vi "Practica3_try2.vi"() -> ()   [LabVIEW 2018]
uses:
  <vilib>/MakerHub/LINX/Public/Peripherals/PWM/PWM Set Duty Cycle 1 Chan.vi
  <vilib>/MakerHub/LINX/Public/Peripherals/Analog/Analog Read 1 Chan.vi
  <vilib>/MakerHub/LINX/Public/Peripherals/Analog/Analog Read N Chans.vi
  <vilib>/MakerHub/LINX/Private/Local IO/LinxAnalogRead.vi
  <vilib>/MakerHub/LINX/Public/Utilities/Check Channel.vi
  <vilib>/MakerHub/LINX/Public/Utilities/Open Serial.vi
  <vilib>/MakerHub/LINX/Public/Sensors/Temperature/TMP3x/TMP35.vi
  <vilib>/MakerHub/LINX/Public/Peripherals/PWM/PWM Set Duty Cycle N Chans.vi
  <vilib>/MakerHub/LINX/Private/Utilties/Generate Error.vi
  <vilib>/MakerHub/LINX/LMH-LINX.lvlib
  <vilib>/MakerHub/LINX/Public/Sensors/Temperature/TMP3x/TMP3x.lvlib
  <vilib>/ptbypt/NI_PtbyPt.lvlib
panel:
  in  "y 3":errorcluster
  in  "y 2":errorcluster
  out "Boolean":bool
  in  "Serial Port":refnum<visa-resource-name>="N/A"
  in  "Temperatura limite":dbl
  out "Thermometer":dbl(slide) scale=0.0..100.0
  in  "y":errorcluster
  out "Color Box 2":u32(colorbox)
  in  "intensidd verde":dbl=0.3
  in  "Temperatur optima(led azul)":dbl=0.25 format="%#_13g"
  in  "stop":bool
  in  "hall":bool
  in  "lm35":bool
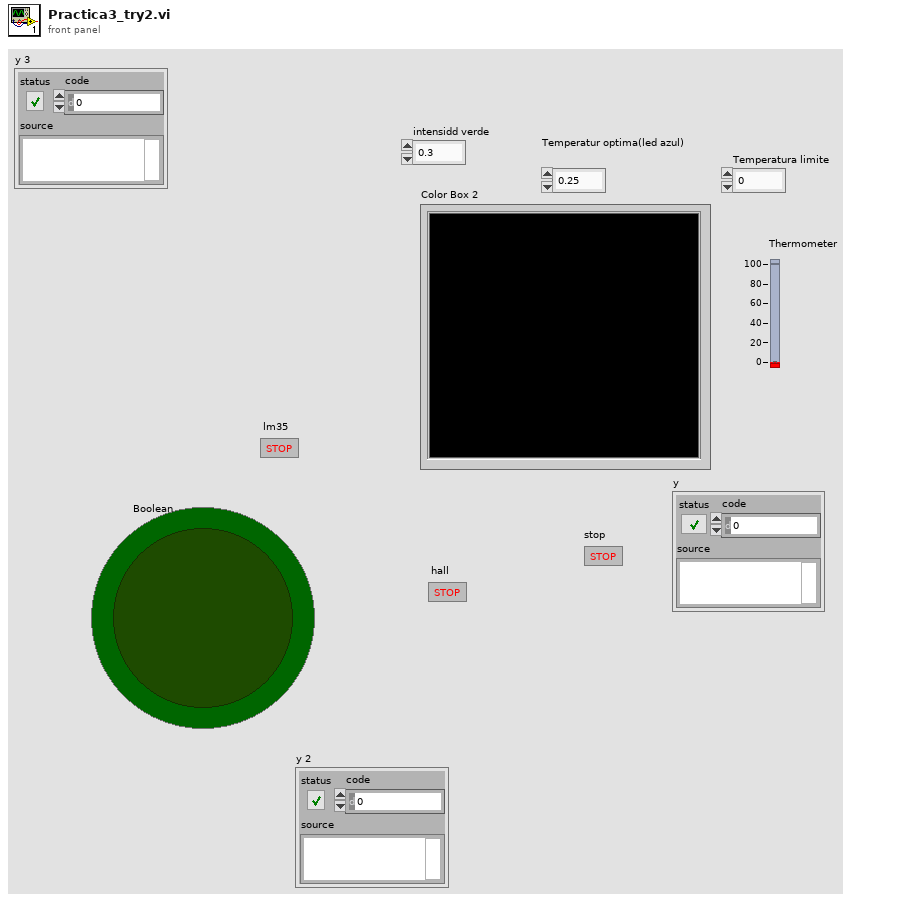
[diagram p1: front panel]
types:
  T1 = typedef "LMH-LINX.lvlib/LINX Ref.ctl" = cluster{"IO":T2, "Interface":T3, "LINX Device Config":T4}
  T2 = typedef "LMH-LINX.lvlib/Platform.ctl" = enum16{"Remote", "Local"}
  T3 = typedef "LMH-LINX.lvlib/Interface.ctl" = enum16{"Serial", "TCP"}
  T4 = typedef "LMH-LINX.lvlib/Device.lvlib/LINX Device Config.ctl" = cluster{"Interface":T3, "COM Port":refnum<visa-resource-name>, "TCP Configuration":T5, "Device Family":u8, "Device ID":u8, "Device Name":string, "TCP Ref":refnum<k5>, "Channels":T6}
  T5 = typedef "LMH-LINX.lvlib/Device.lvlib/TCP Config.ctl" = cluster{"IP Address":string, "Port":u16}
  T6 = typedef "LMH-LINX.lvlib/Channels.ctl" = cluster{"DI":u8[], "DO":u8[], "AI":u8[], "AO":u8[], "PWM":u8[], "QE":u8[], "UART":u8[], "I2C 2":u8[], "SPI":u8[], "CAN":u8[], "Servo":u8[], "AI Ref (V)":dbl, "AI Resolution (Bits)":u8, "AO Ref (V)":dbl, "AO Resolution (Bits)":u8}
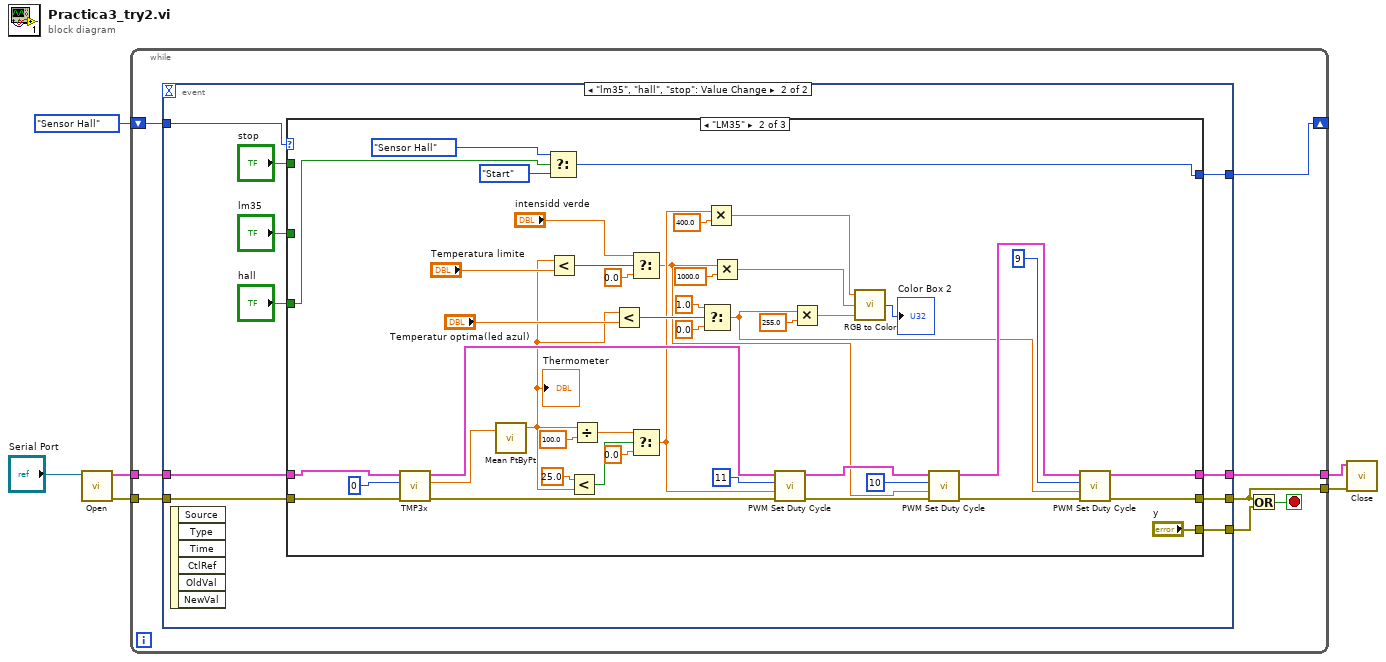
[diagram p0: block diagram]
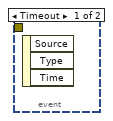
[diagram p2: hidden frame]
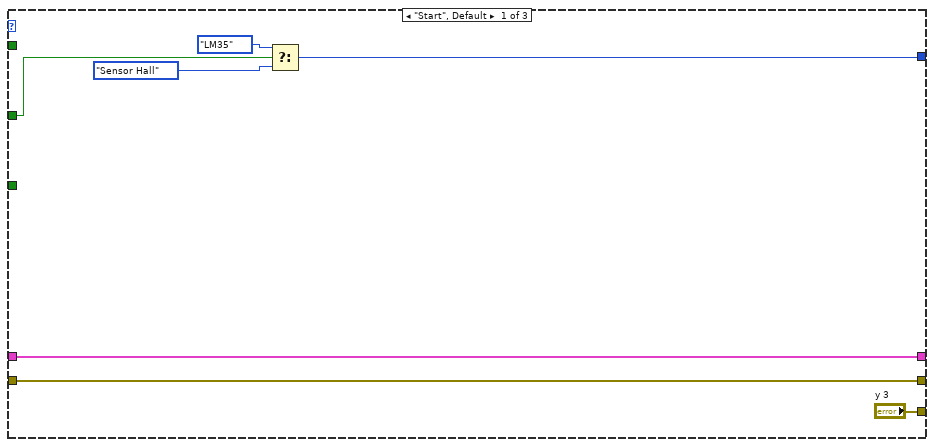
[diagram p3: hidden frame]
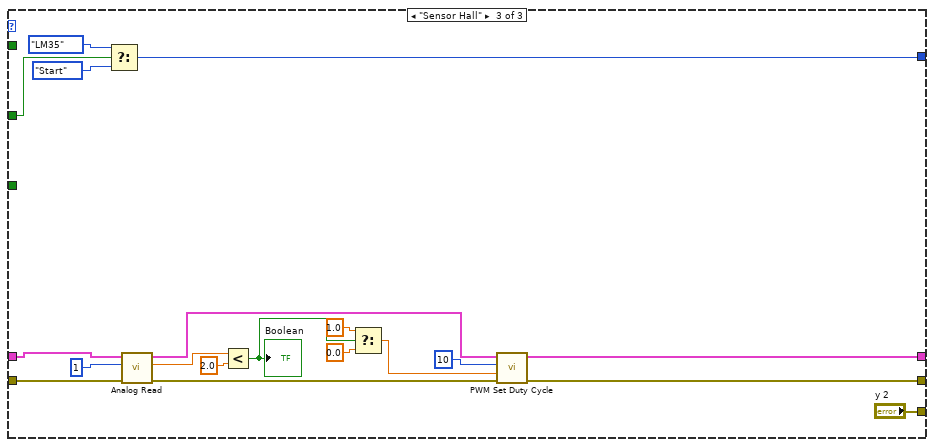
[diagram p4: hidden frame]
diagram:
  n1 = call-poly <vilib>:"Open.vi"("Serial Port"="Serial Port") -> ("Error Out"=w3:errorcluster, "LINX Resource"=w4:T1)  [unwired: 8 in, 1 out]
  n2 = while {
    shift-right: [w14] -> _
    shift-left: enum16{"Start", "LM35", "Sensor Hall"}."Sensor Hall" -> [w13]
    tunnel: w4 -> [w12]
    tunnel: w3 -> [w11]
    tunnel: [w10] -> w2
    tunnel: [w8] -> w1
    stop <- w9 stop-if-true
    n3 = event shown="[1] \"lm35\", \"hall\", \"stop\": Value Change" {
      selector: _ -> [_ _]
      dyn-events: _ -> [_ _]
      timeout: _ -> [_ _]
      tunnel: w13 -> [_ w24]
      tunnel: [_ w20] -> w14
      tunnel: w12 -> [_ w19]
      tunnel: w11 -> [_ w18]
      tunnel: [_ w17] -> w10
      tunnel: [_ w16] -> w8
      tunnel: [_ w15] -> w7
      event Timeout {
        n4 = event-data() -> ()  [unwired: 1 in, 3 out]
      }
      event "lm35", "hall", "stop": Value Change {
        n5 = event-data() -> ()  [unwired: 1 in, 6 out]
        n6 = case shown="\"LM35\"" w24 {
          tunnel: "stop" -> [_ _ _]
          tunnel: "lm35" -> [w28 _ w92]
          tunnel: "hall" -> [_ w75 _]
          tunnel: [w30 w73 w91] -> w20
          tunnel: w19 -> [w27 w36 w77]
          tunnel: w18 -> [w26 w35 w76]
          tunnel: [w27 w34 w80] -> w17
          tunnel: [w26 w33 w79] -> w16
          tunnel: ["y 3" "y" "y 2"] -> w15
          frame "Start", Default {
            n7 = Select(t=enum16{"Start", "LM35", "Sensor Hall"}."LM35", s=w28, f=enum16{"Start", "LM35", "Sensor Hall"}."Sensor Hall") -> (s? t:f=w30:enum16{"Start", "LM35", "Sensor Hall"})
          }
          frame "LM35" {
            n8 = call-poly <vilib>:"TMP3x.vi"("Error In"=w35, "Analog Channel"=u8 0, "LINX Resource"=w36) -> ("Error Out"=w61:errorcluster, "Temp C"=w43:dbl, "LINX Resource"=w60:T1)  [unwired: 6 in]
            n9 = call <vilib>:"Mean PtByPt.vi"("x"=w43) -> ("mean"=w37:dbl)  [unwired: 3 in, 1 out]
            "Thermometer" <- w37
            n10 = Select(t=enum16{"Start", "LM35", "Sensor Hall"}."Sensor Hall", s=w75, f=enum16{"Start", "LM35", "Sensor Hall"}."Start") -> (s? t:f=w73:enum16{"Start", "LM35", "Sensor Hall"})
            n11 = Less?(x=w37, y="Temperatura limite") -> (x < y?=w42:bool)
            n12 = Less?(x=25.0, y=w37) -> (x < y?=w62:bool)
            n13 = Divide(x=w37, y=100.0) -> (x/y=w57:dbl)
            n14 = Less?(x=w37, y="Temperatur optima(led azul)") -> (x < y?=w66:bool)
            n15 = Select(t="intensidd verde", s=w42, f=0.0) -> (s? t:f=w41:dbl)
            n16 = Select(t=w57, s=w62, f=0.0) -> (s? t:f=w52:dbl)
            n17 = Select(t=1.0, s=w66, f=0.0) -> (s? t:f=w44:dbl)
            n18 = Multiply(x=w52, y=400.0) -> (x*y=w47:dbl)
            n19 = Multiply(x=w41, y=1000.0) -> (x*y=w46:dbl)
            n20 = call-poly <vilib>:"PWM Set Duty Cycle.vi"("Error In"=w61, "Duty Cycle (0-1)"=w52, "PWM Channel"=u32 11, "LINX Resource"=w60) -> ("Error Out"=w70:errorcluster, "LINX Resource"=w71:T1)  [unwired: 6 in]
            n21 = Multiply(x=w44, y=255.0) -> (x*y=w49:dbl)
            n22 = call <vilib>:"RGB to Color.vi"("B"=w49, "G"=w46, "R"=w47) -> ("Color"=→"Color Box 2":u32)
            n23 = call-poly <vilib>:"PWM Set Duty Cycle.vi"("Error In"=w70, "Duty Cycle (0-1)"=w41, "PWM Channel"=u8 10, "LINX Resource"=w71) -> ("Error Out"=w68:errorcluster, "LINX Resource"=w69:T1)  [unwired: 6 in]
            n24 = call-poly <vilib>:"PWM Set Duty Cycle.vi"("Error In"=w68, "Duty Cycle (0-1)"=w44, "PWM Channel"=u8 9, "LINX Resource"=w69) -> ("Error Out"=w33:errorcluster, "LINX Resource"=w34:T1)  [unwired: 6 in]
          }
          frame "Sensor Hall" {
            n25 = Select(t=enum16{"Start", "LM35", "Sensor Hall"}."LM35", s=w92, f=enum16{"Start", "LM35", "Sensor Hall"}."Start") -> (s? t:f=w91:enum16{"Start", "LM35", "Sensor Hall"})
            n26 = call-poly <vilib>:"Analog Read.vi"("Error In"=w76, "Analog Channel"=u8 1 ("DI Channel"), "LINX Resource"=w77) -> ("Error Out"=w85:errorcluster, "Voltage"=w82:dbl, "LINX Resource"=w86:T1)  [unwired: 5 in, 1 out]
            n27 = Less?(x=w82, y=2.0) -> (x < y?=w81:bool)
            "Boolean" <- w81
            n28 = Select(t=1.0, s=w81, f=0.0) -> (s? t:f=w84:dbl)
            n29 = call-poly <vilib>:"PWM Set Duty Cycle.vi"("Error In"=w85, "Duty Cycle (0-1)"=w84, "PWM Channel"=u8 10, "LINX Resource"=w86) -> ("Error Out"=w79:errorcluster, "LINX Resource"=w80:T1)  [unwired: 6 in]
          }
        }
      }
    }
    n30 = Or(x=w8, y=w7) -> (x .or. y?=w9:bool)
  }
  n31 = call <vilib>:"Close.vi"("Error In"=w1, "LINX Resource"=w2) -> ()  [unwired: 9 in, 1 out]
